vi "MotorInfo.vi"(6 "error in (no error)":errorcluster, 9 "Motor":string) -> (0 "error out":errorcluster, 3 "Motor out":string, 4 "Axis status":T1)   [LabVIEW 2009]
uses:
  Controls/MotorStatus.ctl
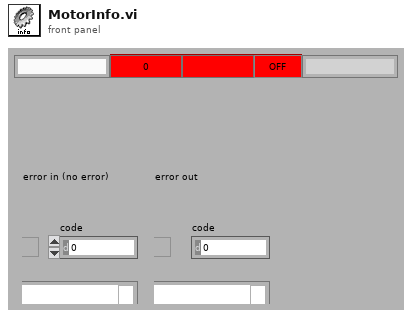
[diagram p1: front panel]
types:
  T1 = typedef "MotorStatus.ctl" = cluster{"Managed?":bool, "Position":i32, "Name":string, "Status":enum16{"OFF", "IDLE", "MOVING", "HOMING"}}
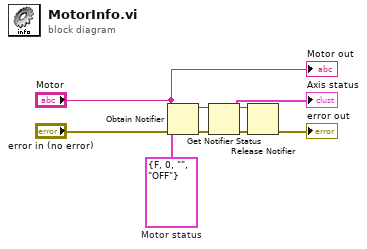
[diagram p0: block diagram]
diagram:
  w2 = T1 {"Managed?"=FALSE, "Position"=0, "Name"="", "Status"=enum."OFF"}  # Motor status
  n1 = Obtain Notifier(name (unnamed)="Motor", notification data type=w2, error in (no error)="error in (no error)") -> (notifier out=w5:refnum<notifier>, error out=w6:errorcluster)  [unwired: 1 in, 1 out]
  n2 = Get Notifier Status(notifier=w5, error in (no error)=w6) -> (notifier out=w8:refnum<notifier>, current notification=→"Axis status":T1, error out=w7:errorcluster)  [unwired: 2 out]
  n3 = Release Notifier(notifier=w8, error in (no error)=w7) -> (error out=→"error out":errorcluster)  [unwired: 3 out]
  "Motor out" <- "Motor"
